vi "Do.vi"(8 "error in (no error)":errorcluster, 10 "Key":string, 11 "Proto in":refnum<class "Proto.lvclass">) -> (0 "error out":errorcluster, 2 "Value":bool, 3 "Proto out":refnum<class "Proto.lvclass">)   [LabVIEW 2020, in "Proto.lvclass"]
uses:
  Proto.lvclass
  Proto.lvclass/Proto.ctl
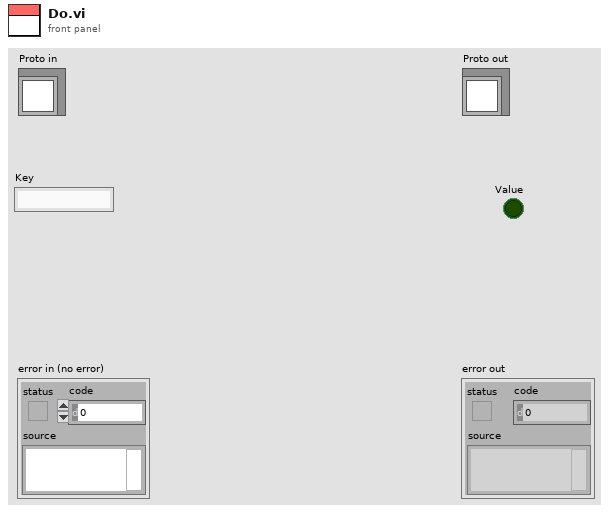
[diagram p1: front panel]
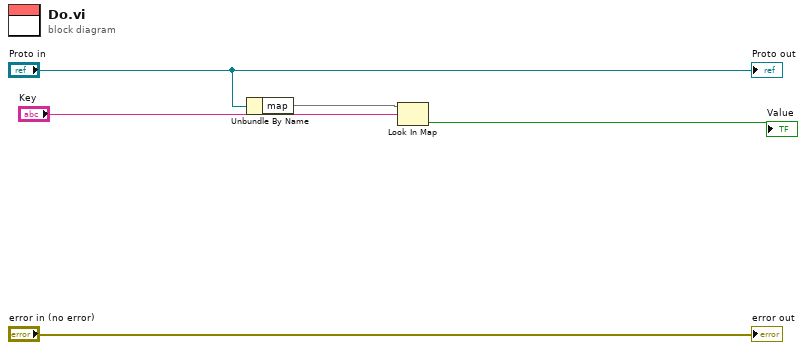
[diagram p0: block diagram]
diagram:
  n1 = Unbundle By Name("Proto in") -> ("map"=w3:map{string, bool})
  n2 = Look In Map(map=w3, key="Key") -> (value=→"Value":bool)  [unwired: 1 in, 1 out]
  "error out" <- "error in (no error)"
  "Proto out" <- "Proto in"
